vi "Check ECAT Reconfig.vi"(2 "R/W Case":T34, 7 "RT Data in":T1={"Device ref"=0, "Scan Period (uSec)"=10000, "Device Channels"={"Status"={"BD Refs"=[], "Length"=0, "FIFO Index"=0, "Data"=[]}, "Command"={"BD Refs"=[], "Data"=[], "Length"=0, "FIFO Index"=0}}, "Local Chassis"=[], "EtherCAT Masters"=[], "Async"={"Status"=refnum, "Command"=refnum, "Input FIFO"=refnum, "Input FIFO buffer"=[], "Output FIFO"=refnum, "Output FIFO buffer"=[], "Async VI Ref"=refnum}, "ECAT Reconfig"={"Reconfig Module Found"=FALSE, "VI Ref"=refnum, "Status"=refnum}, "Device Error"={"status"=FALSE, "code"=0, "source"=""}, "DeviceName"="", "PCLSync?"=FALSE} {"Device Channels"."Status"."BD Refs"."Data Reference" format="%.0x"; "Device Channels"."Command"."BD Refs"."Data Reference" format="%.0x"; "Local Chassis"."FPGA"."VS ref" format="%.0x"; "Local Chassis"."RSI Modules"."VS ref" format="%.0x"; "Local Chassis"."VS ref" format="%.0x"; "Device ref" format="%.0x"; "EtherCAT Masters"."DS402 Drive ECAT Slaves"."VS ref" format="%.0x"; "EtherCAT Masters"."REM IO ECAT Slaves"."VS ref" format="%.0x"; "EtherCAT Masters"."Generic EtherCAT Slaves"."VS ref" format="%.0x"; "EtherCAT Masters"."VS ref" format="%.0x"; "EtherCAT Masters"."EtherCAT Slaves"."FPGA"."VS ref" format="%.0x"; "EtherCAT Masters"."EtherCAT Slaves"."RSI Modules"."VS ref" format="%.0x"; "EtherCAT Masters"."EtherCAT Slaves"."VS ref" format="%.0x"}) -> (8 "RT Data out":T1={"Device ref"=0, "Scan Period (uSec)"=10000, "Device Channels"={"Status"={"BD Refs"=[], "Length"=0, "FIFO Index"=0, "Data"=[]}, "Command"={"BD Refs"=[], "Data"=[], "Length"=0, "FIFO Index"=0}}, "Local Chassis"=[], "EtherCAT Masters"=[], "Async"={"Status"=refnum, "Command"=refnum, "Input FIFO"=refnum, "Input FIFO buffer"=[], "Output FIFO"=refnum, "Output FIFO buffer"=[], "Async VI Ref"=refnum}, "ECAT Reconfig"={"Reconfig Module Found"=FALSE, "VI Ref"=refnum, "Status"=refnum}, "Device Error"={"status"=FALSE, "code"=0, "source"=""}, "DeviceName"="", "PCLSync?"=FALSE} {"Device Channels"."Status"."BD Refs"."Data Reference" format="%.0x"; "Device Channels"."Command"."BD Refs"."Data Reference" format="%.0x"; "Local Chassis"."FPGA"."VS ref" format="%.0x"; "Local Chassis"."RSI Modules"."VS ref" format="%.0x"; "Local Chassis"."VS ref" format="%.0x"; "Device ref" format="%.0x"; "EtherCAT Masters"."DS402 Drive ECAT Slaves"."VS ref" format="%.0x"; "EtherCAT Masters"."REM IO ECAT Slaves"."VS ref" format="%.0x"; "EtherCAT Masters"."Generic EtherCAT Slaves"."VS ref" format="%.0x"; "EtherCAT Masters"."VS ref" format="%.0x"; "EtherCAT Masters"."EtherCAT Slaves"."FPGA"."VS ref" format="%.0x"; "EtherCAT Masters"."EtherCAT Slaves"."RSI Modules"."VS ref" format="%.0x"; "EtherCAT Masters"."EtherCAT Slaves"."VS ref" format="%.0x"}, 13 "ECAT Reconfig?":bool)   [LabVIEW 2016, in "Scan Engine Custom Device.lvlib"]
uses:
  Scan Engine Custom Device.lvlib
  Type Defs/RW Case.ctl
  Type Defs/RT Data.ctl
  <vilib>/NI Veristand/Custom Device API/Custom Device Item Ref.ctl
  Type Defs/Device Channels.ctl
  Type Defs/Output Data.ctl
  <vilib>/NI Veristand/Custom Device API/Block Data Reference.ctl
  <vilib>/NI Veristand/Custom Device API/Data Reference.ctl
  Type Defs/Input Data.ctl
  Type Defs/Local Chassis Data.ctl
  Type Defs/RSI Module Data.ctl
  Type Defs/Open Module IOVs.ctl
  Modules.lvlibp/RSI Module/RSI Module.lvclass
  Modules.lvlibp/RSI Module/Module Models.ctl
  Modules.lvlibp/RSI Module/Channel Type.ctl
  Type Defs/Module Config Data.ctl
  Type Defs/Mixed IO.ctl
  Type Defs/FPGA Data.ctl
  Type Defs/UDV Data.ctl
  Type Defs/UDV Data Type.ctl
  Type Defs/FXP Config.ctl
  Type Defs/Mod Size Indexes.ctl
  Type Defs/EtherCAT Master Data.ctl
  Type Defs/EtherCAT Slave Data.ctl
  Type Defs/Generic ECAT Slave RT-Data-Array.ctl
  Type Defs/Generic ECAT Slave Data Cluster.ctl
  Type Defs/Generic ECAT Slave IOV Cluster.ctl
  Type Defs/REM IO ECAT Slave RT-Data-Array.ctl
  Type Defs/REM IO ECAT Slave Data Cluster.ctl
  Type Defs/REM IO ECAT Slave IOV Cluster.ctl
  Type Defs/DS402 Drive ECAT Slave RT-Data-Array.ctl
  Type Defs/DS402 Drive ECAT Slave Data Cluster.ctl
  Type Defs/DS402 Drive ECAT Slave IOV Cluster.ctl
  Type Defs/DS402 Drive ECAT Slave Action IOV Cluster.ctl
  Type Defs/Async Data.ctl
  Type Defs/Async Status.ctl
  Type Defs/Async State.ctl
  Type Defs/Async Command.ctl
  Type Defs/ECAT Reconfig Data.ctl
  Type Defs/ECAT Reconfig Status.ctl
  Type Defs/ECAT Reconfig State.ctl
  Utility/Set Error.vi
  Globals/Error Strings.vi
  <vilib>/NI Veristand/Custom Device API/Custom Device API.lvlib
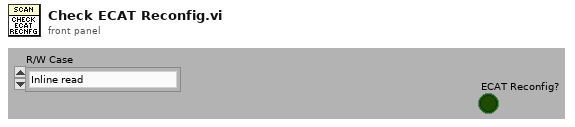
[diagram p1: front panel]
types:
  T1 = typedef "Scan Engine Custom Device.lvlib/RT Data.ctl" = cluster{"Device ref":T2, "Scan Period (uSec)":u32, "Device Channels":T3, "Local Chassis":T8[], "EtherCAT Masters":T20[], "Async":T32, "ECAT Reconfig":T33, "Device Error":errorcluster, "DeviceName":string, "PCLSync?":bool}
  T2 = typedef "Custom Device API.lvlib/Custom Device Item Ref.ctl" = u64
  T3 = typedef "Scan Engine Custom Device.lvlib/Device Channels.ctl" = cluster{"Status":T4, "Command":T7}
  T4 = typedef "Scan Engine Custom Device.lvlib/Output Data.ctl" = cluster{"BD Refs":T5[], "Length":i32, "FIFO Index":i32, "Data":dbl[]}
  T5 = typedef "Custom Device API.lvlib/Block Data Reference.ctl" = cluster{"Data Reference":T6, "Offset":u64, "Length":u64}
  T6 = typedef "Custom Device API.lvlib/Data Reference.ctl" = i32
  T7 = typedef "Scan Engine Custom Device.lvlib/Input Data.ctl" = cluster{"BD Refs":T5[], "Data":dbl[], "Length":i32, "FIFO Index":i32}
  T8 = typedef "Scan Engine Custom Device.lvlib/Local Chassis Data.ctl" = cluster{"VS ref":T2, "RSI Modules":T9[], "FPGA":T15[], "Input Mod Size Idxs":T19, "Output Modules":i32[], "MixedIO Mod Size Idxs":T19}
  T9 = typedef "Scan Engine Custom Device.lvlib/RSI Module Data.ctl" = cluster{"VS ref":T2, "IOV ref":refnum<k21>, "Open Mod refs":T10, "Module DVR":refnum<data-value>, "Slot":u32, "Model":T11, "Channel Type":T12, "EtherCAT?":bool, "CDInput Data":T7, "CDOutput Data":T4, "Module Config Data":T13, "Mixed IO":T14}
  T10 = typedef "Scan Engine Custom Device.lvlib/Open Module IOVs.ctl" = cluster{"Analog Read":refnum<k21>, "Digital Read":refnum<k21>, "Analog Write":refnum<k21>, "Digital Write":refnum<k21>}
  T11 = typedef "Modules.lvlibp/RSI Module.lvclass/Module Models.ctl" = enum16{"Empty", "NI 9201", "NI 9203", "NI 9205", "NI 9206", "NI 9207", "NI 9208", "NI 9211", "NI 9212", "NI 9213", "NI 9214", "NI 9215", "NI 9217", "NI 9219", "NI 9220", "NI 9221", "NI 9222", "NI 9223", "NI 9225", "NI 9227", "NI 9229", "NI 9233", "NI 9234", "NI 9235", "NI 9236", "NI 9237", "NI 9239", "NI 9242", "NI 9244", "NI 9263", "NI 9264", "NI 9265", "NI 9269", "NI 9375", "NI 9401", "NI 9402", "NI 9403", "NI 9411", "NI 9421", "NI 9422", "NI 9423", "NI 9425", "NI 9426", "NI 9435", "NI 9437", "NI 9472", "NI 9474", "NI 9475", "NI 9476", "NI 9477", "NI 9478", "NI 9481", "NI 9482", "NI 9485"}
  T12 = typedef "Modules.lvlibp/RSI Module.lvclass/Channel Type.ctl" = enum16{"Analog", "Digital"}
  T13 = typedef "Scan Engine Custom Device.lvlib/Module Config Data.ctl" = cluster{"Configurable?":bool, "Config Block Data Refs":T5[], "Config Data DVR":refnum<data-value>, "Previous Values":dbl[], "Local Reconfig VI Ref":refnum<vi>}
  T14 = typedef "Scan Engine Custom Device.lvlib/Mixed IO.ctl" = cluster{"Input Channel Indices":i32[], "Input Buffer":dbl[]}
  T15 = typedef "Scan Engine Custom Device.lvlib/FPGA Data.ctl" = cluster{"VS ref":T2, "IOV ref":refnum<k21>, "FPGA Target":enum16{"Local", "EtherCAT"}, "Product Code":u32, "Bitfile Signature":string, "Bitfile Path (RT)":path, "FPGA Session":u32, "Input Data":T7, "Output Data":T4, "UDVs":cluster{"From FPGA":T16[], "To FPGA":T16[]}}
  T16 = typedef "Scan Engine Custom Device.lvlib/UDV Data.ctl" = cluster{"VS ref":T2, "IOV Ref":refnum<k21>, "Name":string, "UDV Data Type":T17, "Supported Type?":bool, "FXP Config":T18, "FXP VI Ref":refnum<vi>}
  T17 = typedef "Scan Engine Custom Device.lvlib/UDV Data Type.ctl" = enum16{"Boolean", "Fixed Point", "Int8", "Int16", "Int32", "Int64", "U32 Bit Field", "UInt8", "UInt16", "UInt32", "UInt64", "Other"}
  T18 = typedef "Scan Engine Custom Device.lvlib/FXP Config.ctl" = cluster{"signed":bool, "size":u32, "integersize":i32}
  T19 = typedef "Scan Engine Custom Device.lvlib/Mod Size Indexes.ctl" = cluster{"4":i32[], "8":i32[], "16":i32[], "32":i32[], "other":i32[]}
  T20 = typedef "Scan Engine Custom Device.lvlib/EtherCAT Master Data.ctl" = cluster{"VS ref":T2, "IOV ref":refnum<k21>, "Master ID":u32, "Cyclic Data Bandwidth":u32, "EtherCAT Slaves":T21[], "Generic EtherCAT Slaves":T22, "REM IO ECAT Slaves":T25, "DS402 Drive ECAT Slaves":T28}
  T21 = typedef "Scan Engine Custom Device.lvlib/EtherCAT Slave Data.ctl" = cluster{"VS ref":T2, "IOV ref":refnum<k21>, "Position Address":u16, "RSI Modules":T9[], "FPGA":T15[], "Input Mod Size Idxs":T19, "Output Modules":i32[], "MixedIO Mod Size Idxs":T19}
  T22 = typedef "Scan Engine Custom Device.lvlib/Generic ECAT Slave RT-Data-Array.ctl" = T23[]
  T23 = typedef "Scan Engine Custom Device.lvlib/Generic ECAT Slave Data Cluster.ctl" = cluster{"VS ref":T2, "IOV ref":refnum<k21>, "Position Address":u16, "I/O Imput Vars ":T24[], "I/O Output Vars":T24[], "I/O Input Data":T7, "I/O Output Data":T4}
  T24 = typedef "Scan Engine Custom Device.lvlib/Generic ECAT Slave IOV Cluster.ctl" = cluster{"VS ref":T2, "IOV Ref":refnum<k21>, "Name":string, "UDV Data Type":T17}
  T25 = typedef "Scan Engine Custom Device.lvlib/REM IO ECAT Slave RT-Data-Array.ctl" = T26[]
  T26 = typedef "Scan Engine Custom Device.lvlib/REM IO ECAT Slave Data Cluster.ctl" = cluster{"VS ref":T2, "IOV ref":refnum<k21>, "Position Address":u16, "I/O Imput Vars ":T27[], "I/O Output Vars":T27[], "I/O Input Data":T7, "I/O Output Data":T4}
  T27 = typedef "Scan Engine Custom Device.lvlib/REM IO ECAT Slave IOV Cluster.ctl" = cluster{"VS ref":T2, "IOV Ref":refnum<k21>, "Name":string, "UDV Data Type":T17, "Scaling Factor":dbl}
  T28 = typedef "DS402 Drive ECAT Slave RT-Data-Array.ctl" = T29[]
  T29 = typedef "Scan Engine Custom Device.lvlib/DS402 Drive ECAT Slave Data Cluster.ctl" = cluster{"VS ref":T2, "IOV ref":refnum<k21>, "Position Address":u16, "I/O Input Vars ":T30[], "I/O Output Vars":T30[], "I/O Input Data":T7, "I/O Output Data":T4, "DS402 IOV":T31}
  T30 = typedef "Scan Engine Custom Device.lvlib/DS402 Drive ECAT Slave IOV Cluster.ctl" = cluster{"VS ref":T2, "IOV Ref":refnum<k21>, "Name":string, "UDV Data Type":T17, "Scaling Factor":dbl, "IOV":bool, "VS data Index":i32}
  T31 = typedef "Scan Engine Custom Device.lvlib/DS402 Drive ECAT Slave Action IOV Cluster.ctl" = cluster{"Control Word":refnum<k21>, "Status Word":refnum<k21>}
  T32 = typedef "Scan Engine Custom Device.lvlib/Async Data.ctl" = cluster{"Status":refnum<queue>, "Command":refnum<queue>, "Input FIFO":refnum<k33>, "Input FIFO buffer":dbl[], "Output FIFO":refnum<k33>, "Output FIFO buffer":dbl[], "Async VI Ref":refnum<vi>}
  T33 = typedef "Scan Engine Custom Device.lvlib/ECAT Reconfig Data.ctl" = cluster{"Reconfig Module Found":bool, "VI Ref":refnum<vi>, "Status":refnum<queue>}
  T34 = typedef "Scan Engine Custom Device.lvlib/RW Case.ctl" = enum16{"Inline read", "Inline write", "Async - Inline loop read", "Async - Inline loop write", "Async loop (read/write)"}
  T35 = typedef "Scan Engine Custom Device.lvlib/Async State.ctl" = enum16{"Not running", "Waiting on start cmd", "Running", "Paused", "Stopped"}
  T36 = typedef "Scan Engine Custom Device.lvlib/ECAT Reconfig State.ctl" = enum16{"Not running", "Waiting to Start", "Started", "Running"}
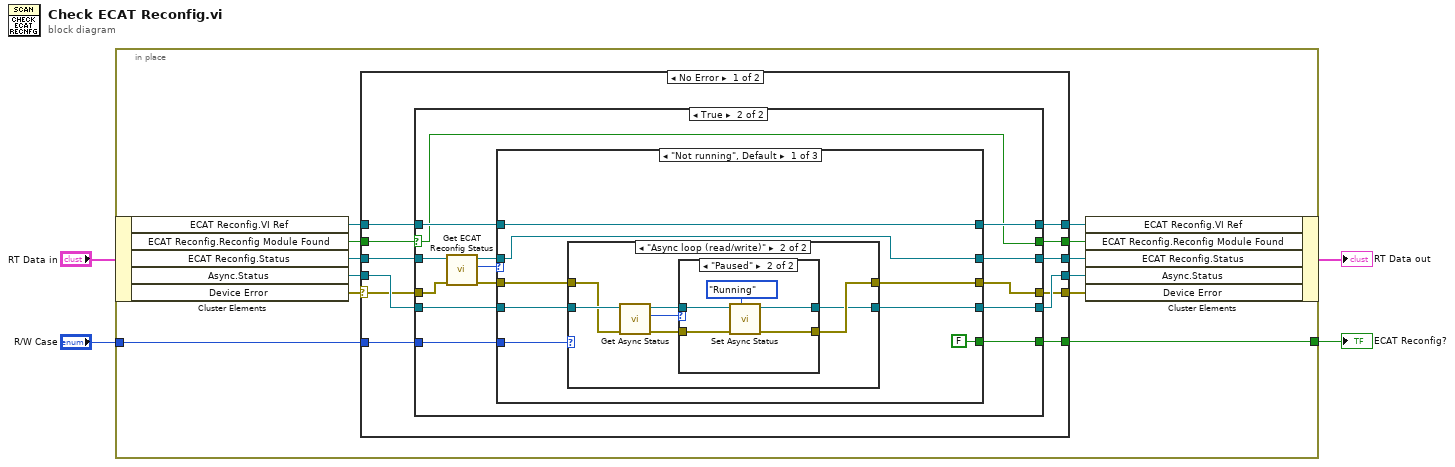
[diagram p0: block diagram]
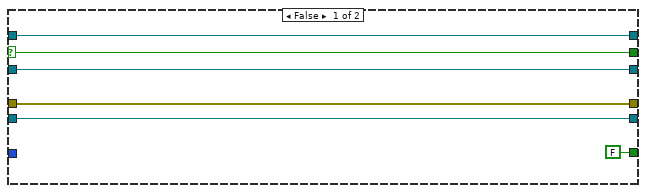
[diagram p2: hidden frame]
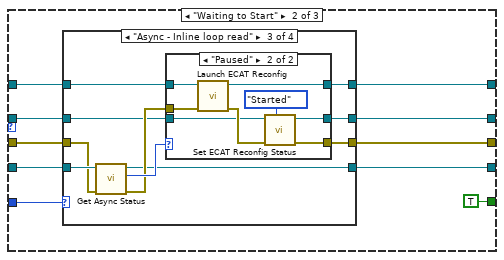
[diagram p5: hidden frame]
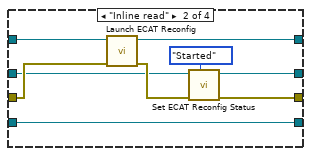
[diagram p7: hidden frame]
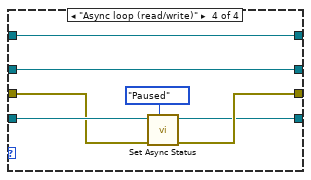
[diagram p9: hidden frame]
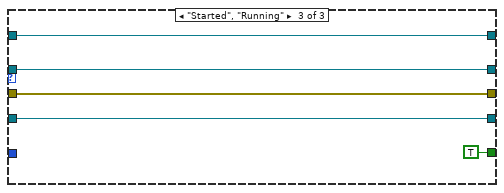
[diagram p10: hidden frame]
diagram:
  n1 = in-place {
    in-place-border: "R/W Case" -> [w16]
    in-place-border: [w13] -> w3
    n2 = in-place-cluster #1("RT Data in") -> ("ECAT Reconfig.VI Ref"=w15:refnum<vi>, "ECAT Reconfig.Reconfig Module Found"=w12:bool, "ECAT Reconfig.Status"=w11:refnum<queue>, "Async.Status"=w8:refnum<queue>, "Device Error"=w5:errorcluster)
    n3 = case shown="No Error" w5 {
      selector: w5 -> [w17 w129]
      tunnel: w16 -> [w28 _]
      tunnel: w15 -> [w27 w133]
      tunnel: [w26 w133] -> w14
      tunnel: [w25 _] -> w13
      tunnel: w12 -> [w24 w132]
      tunnel: w11 -> [w23 w131]
      tunnel: [w22 w131] -> w10
      tunnel: [w21 w132] -> w9
      tunnel: w8 -> [w20 w130]
      tunnel: [w19 w130] -> w7
      tunnel: [w18 w129] -> w6
      frame No Error {
        n4 = case shown="True" w24 {
          selector: w24 -> [w31 w36]
          tunnel: w23 -> [w33 w48]
          tunnel: w17 -> [w34 w47]
          tunnel: w28 -> [_ w43]
          tunnel: w20 -> [w29 w42]
          tunnel: w27 -> [w32 w41]
          tunnel: [w34 w40] -> w18
          tunnel: [w32 w39] -> w26
          tunnel: [w33 w38] -> w22
          tunnel: [FALSE w37] -> w25
          tunnel: [w31 w36] -> w21
          tunnel: [w29 w35] -> w19
          frame False {
          }
          frame True {
            n5 = call "Get ECAT Reconfig Status.vi"("error in (no error)"=w47, "Status in"=w48) -> ("error out"=w44:errorcluster, "State"=w46:T36, "Status out"=w45:refnum<queue>)  [unwired: 7 in]
            n6 = case shown="\"Not running\", Default" w46 {
              tunnel: w45 -> [w55 w75 w125]
              tunnel: w44 -> [w51 w80 w128]
              tunnel: w43 -> [w53 w82 _]
              tunnel: w42 -> [w52 w81 w124]
              tunnel: w41 -> [w56 w79 w126]
              tunnel: [w50 w78 w128] -> w40
              tunnel: [w56 w76 w126] -> w39
              tunnel: [w55 w74 w125] -> w38
              tunnel: [FALSE TRUE TRUE] -> w37
              tunnel: [w49 w73 w124] -> w35
              frame "Not running", Default {
                n7 = case shown="\"Async loop (read/write)\"" w53 {
                  tunnel: w52 -> [w57 w65]
                  tunnel: w51 -> [w58 w64]
                  tunnel: [w58 w60] -> w50
                  tunnel: [w57 w59] -> w49
                  frame Default {
                  }
                  frame "Async loop (read/write)" {
                    n8 = call "Get Async Status.vi"("error in (no error)"=w64, "Status in"=w65) -> ("error out"=w62:errorcluster, "State"=w63:T35, "Status out"=w61:refnum<queue>)  [unwired: 7 in]
                    n9 = case shown="\"Paused\"" w63 {
                      tunnel: w62 -> [w67 w72]
                      tunnel: w61 -> [w66 w71]
                      tunnel: [w67 w69] -> w60
                      tunnel: [w66 w68] -> w59
                      frame Default {
                      }
                      frame "Paused" {
                        n10 = call "Set Async Status.vi"("State"=Async_State."Running", "error in (no error)"=w72, "Status in"=w71) -> ("error out"=w69:errorcluster, "Status out"=w68:refnum<queue>)  [unwired: 7 in]
                      }
                    }
                  }
                }
              }
              frame "Waiting to Start" {
                n11 = case shown="\"Async - Inline loop read\"" w82 {
                  tunnel: w81 -> [w83 w89 w105 w123]
                  tunnel: w80 -> [w86 w95 w104 w121]
                  tunnel: w79 -> [w85 w88 w102 w120]
                  tunnel: [w86 w93 w100 w118] -> w78
                  tunnel: [w85 w87 w99 w120] -> w76
                  tunnel: w75 -> [w84 w91 w98 w119]
                  tunnel: [w84 w92 w97 w119] -> w74
                  tunnel: [w83 w89 w96 w117] -> w73
                  frame Default {
                  }
                  frame "Inline read" {
                    n12 = call "Launch ECAT Reconfig.vi"("error in (no error)"=w95, "ECAT Reconfig VI Ref in"=w88) -> ("error out"=w94:errorcluster, "ECAT Reconfig VI Ref out"=w87:refnum<vi>)  [unwired: 8 in]
                    n13 = call "Set ECAT Reconfig Status.vi"("State"=ECAT_Reconfig_State."Started", "error in (no error)"=w94, "Status in"=w91) -> ("error out"=w93:errorcluster, "Status out"=w92:refnum<queue>)  [unwired: 7 in]
                  }
                  frame "Async - Inline loop read" {
                    n14 = call "Get Async Status.vi"("error in (no error)"=w104, "Status in"=w105) -> ("error out"=w101:errorcluster, "State"=w103:T35, "Status out"=w96:refnum<queue>)  [unwired: 7 in]
                    n15 = case shown="\"Paused\"" w103 {
                      tunnel: w102 -> [w106 w110]
                      tunnel: w101 -> [w108 w116]
                      tunnel: [w108 w114] -> w100
                      tunnel: [w106 w109] -> w99
                      tunnel: w98 -> [w107 w113]
                      tunnel: [w107 w112] -> w97
                      frame Default {
                      }
                      frame "Paused" {
                        n16 = call "Launch ECAT Reconfig.vi"("error in (no error)"=w116, "ECAT Reconfig VI Ref in"=w110) -> ("error out"=w115:errorcluster, "ECAT Reconfig VI Ref out"=w109:refnum<vi>)  [unwired: 8 in]
                        n17 = call "Set ECAT Reconfig Status.vi"("State"=ECAT_Reconfig_State."Started", "error in (no error)"=w115, "Status in"=w113) -> ("error out"=w114:errorcluster, "Status out"=w112:refnum<queue>)  [unwired: 7 in]
                      }
                    }
                  }
                  frame "Async loop (read/write)" {
                    n18 = call "Set Async Status.vi"("State"=Async_State."Paused", "error in (no error)"=w121, "Status in"=w123) -> ("error out"=w118:errorcluster, "Status out"=w117:refnum<queue>)  [unwired: 7 in]
                  }
                }
              }
              frame "Started", "Running" {
              }
            }
          }
        }
      }
      frame Error {
      }
    }
    n19 = in-place-cluster #1("ECAT Reconfig.VI Ref"=w14, "ECAT Reconfig.Reconfig Module Found"=w9, "ECAT Reconfig.Status"=w10, "Async.Status"=w7, "Device Error"=w6) -> (→"RT Data out":T1)
  }
  "ECAT Reconfig?" <- w3
